vi "Configure.vi"(8 "error in (no error)":errorcluster, 10 "ConfigRef In":T1, 11 "Power Meter in":refnum<class "Power Meter.lvclass">) -> (0 "error out":errorcluster, 3 "Power Meter out":refnum<class "Power Meter.lvclass">)   [LabVIEW 2015, in "Power Meter.lvclass"]
uses:
  Power Meter.lvclass
  <vilib>/Utility/config.llb/Config Data RefNum.ctl
  <vilib>/Utility/config.llb/NI_LVConfig.lvlib
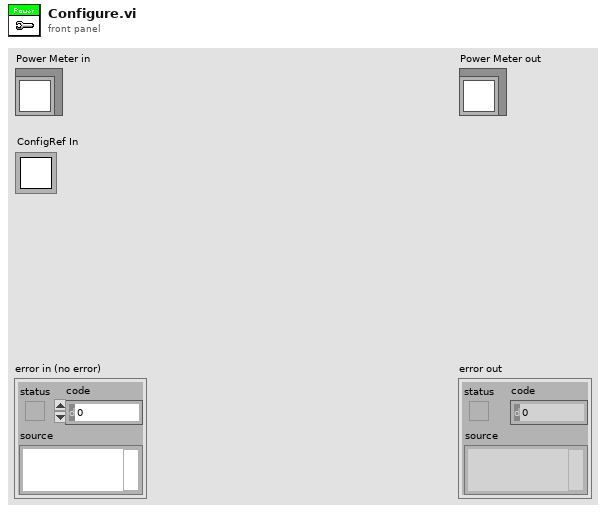
[diagram p1: front panel]
types:
  T1 = typedef "NI_LVConfig.lvlib/Config Data RefNum.ctl" = refnum<k1>
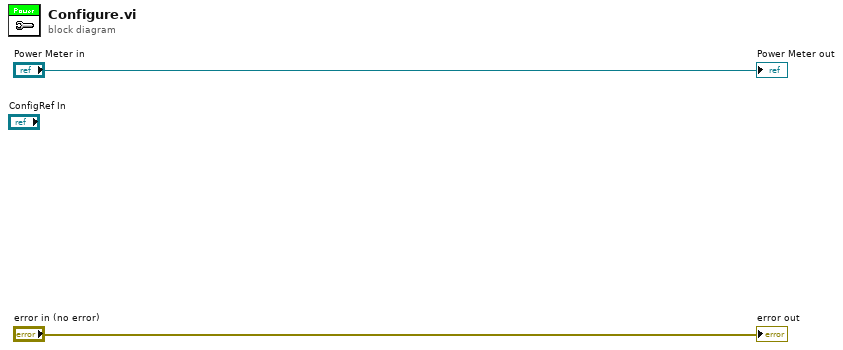
[diagram p0: block diagram]
diagram:
  "error out" <- "error in (no error)"
  "Power Meter out" <- "Power Meter in"
